vi "udp desktop.vi"() -> ()   [LabVIEW 2021]
panel:
  in  "?":bool
  in  "Port":dbl
  in  "IP":string
  in  "Data":string
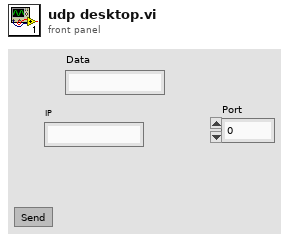
[diagram p1: front panel]
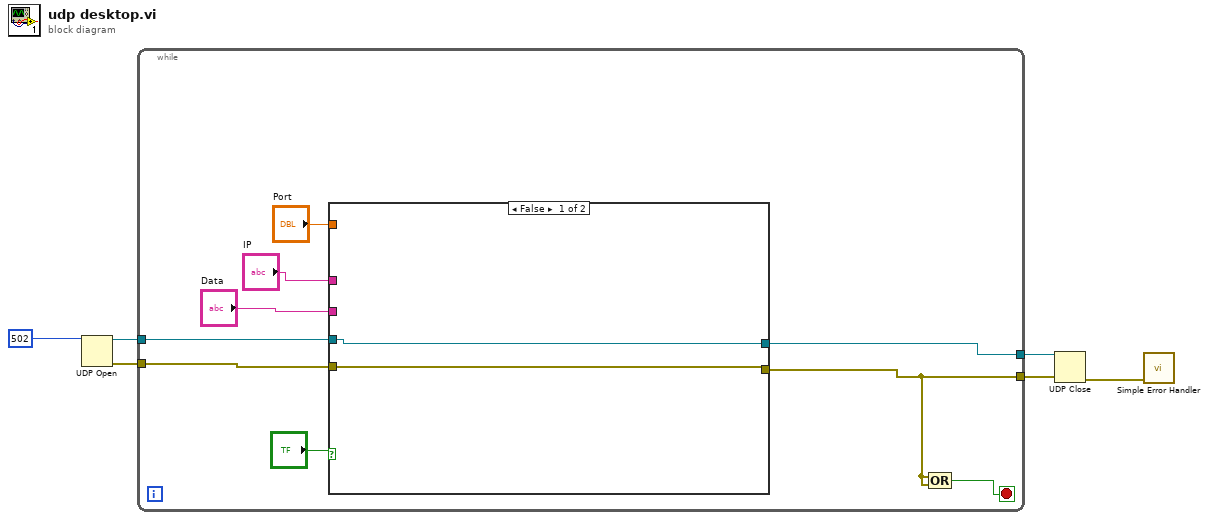
[diagram p0: block diagram]
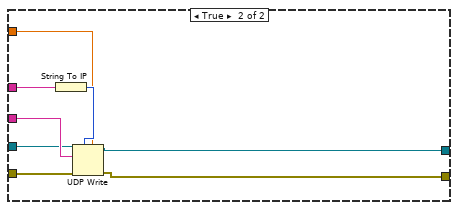
[diagram p2: hidden frame]
diagram:
  n1 = UDP Open(11:502) -> (port=w2:refnum<k16>, 0:w5:errorcluster)  [unwired: 4 in, 1 out]
  n2 = while {
    tunnel: [w7] -> w4
    tunnel: w5 -> [w14]
    tunnel: w2 -> [w11]
    tunnel: [w10] -> w1
    stop <- w9 stop-if-true
    n3 = case shown="False" "?" {
      tunnel: w14 -> [w16 w25]
      tunnel: [w16 w24] -> w7
      tunnel: "IP" -> [_ w23]
      tunnel: "Data" -> [_ w21]
      tunnel: w11 -> [w17 w20]
      tunnel: [w17 w19] -> w10
      tunnel: "Port" -> [_ w18]
      frame False {
      }
      frame True {
        n4 = String To IP(1:w23) -> (0:w22:u32)
        n5 = UDP Write(address=w22, port or service name=w18, connection ID=w20, data in=w21, 8:w25) -> (error out=w24:errorcluster, 3:w19:refnum<k16>)  [unwired: 1 in]
      }
    }
    n6 = Compound Arithmetic op=OR(w7, w7) -> (w9:bool)
  }
  n7 = UDP Close(connection ID=w1, 8:w4) -> (error out=w3:errorcluster)  [unwired: 1 out]
  n8 = call <vilib>:"Simple Error Handler.vi"("error in (no error)"=w3) -> ()  [unwired: 4 in, 5 out]
